vi "GetMessage.vi"(0 "reference in":refnum<class "Colleague.lvclass">, 2 "Sender":string, 5 "error in (no error)":errorcluster, 8 "Message":string) -> (14 "reference out":refnum<class "Colleague.lvclass">, 19 "error out":errorcluster)   [LabVIEW 2013, in "Colleague.lvclass"]
uses:
  Colleague.lvclass
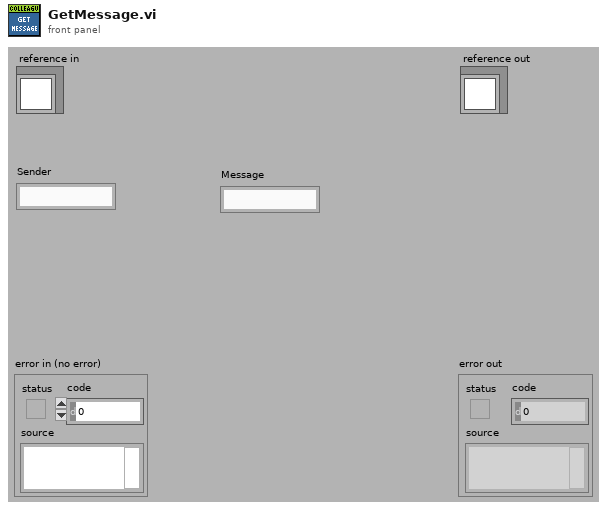
[diagram p1: front panel]
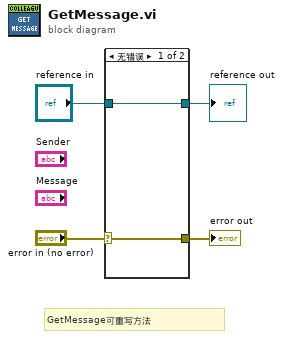
[diagram p0: block diagram]
diagram:
  # "GetMessage可重写方法"
  n1 = case shown="无错误" "error in (no error)" {
    selector: "error in (no error)" -> [w5 w8]
    tunnel: [w5 w8] -> w3
    tunnel: [w6 w7] -> w1
    tunnel: "reference in" -> [w6 w7]
    frame No Error {
      # "GetMessage可重写方法"
    }
    frame Error {
    }
  }
  "error out" <- w3
  "reference out" <- w1
